vi "Load Plugin.vi"(6 "timeout (ms)":i32=5000, 8 "error in":errorcluster, 9 "Plugin Path":string, 10 "Plugin Name":string, 11 "gRPC ID in":T1) -> (0 "error out":errorcluster, 3 "gRPC ID out":T1)   [LabVIEW 2021, in "CIFPluginLoaderClientWrapper.lvlib"]
uses:
  CIFPluginLoaderClientWrapper.lvlib
  <vilib>/gRPC/LabVIEW gRPC Library/Shared/grpcId.ctl
  CIF_PluginLoader_client/RPC Messages/cif_pluginloader_LoadPluginRequest.ctl
  CIF_PluginLoader_client/CIF_PluginLoader_client.lvlib
  <vilib>/gRPC/LabVIEW gRPC Library/grpc-lvsupport-release.lvlib
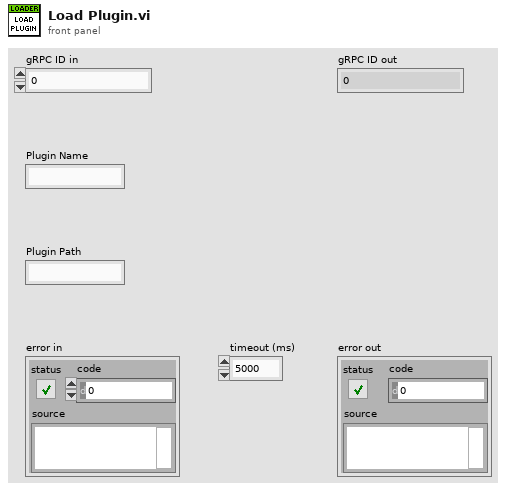
[diagram p1: front panel]
types:
  T1 = typedef "grpc-lvsupport-release.lvlib/grpcId.ctl" = u64
  T2 = typedef "CIF_PluginLoader_client.lvlib/cif_pluginloader_LoadPluginRequest.ctl" = cluster{"plugin_name":string, "path":string}
  T3 = typedef "CIF_PluginLoader_client.lvlib/cif_pluginloader_LoadPluginResponse.ctl" = cluster{"status":T4}
  T4 = typedef "CIF_PluginLoader_client.lvlib/cif_common_Status.ctl" = cluster{"code":i32, "message":string}
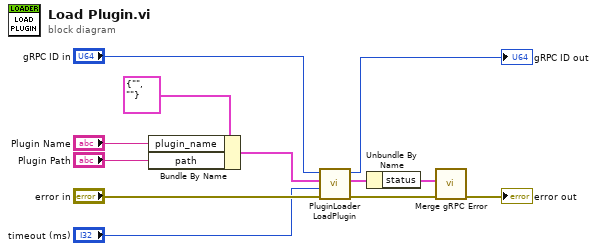
[diagram p0: block diagram]
diagram:
  n1 = Bundle By Name(cluster=T2 {"plugin_name"="", "path"=""} ("Request Data"), "plugin_name"="Plugin Name", "path"="Plugin Path") -> (w3:T2)
  n2 = call "PluginLoader LoadPlugin.vi"("error in"="error in", "timeout (ms)"="timeout (ms)", "Request Data"=w3, "gRPC ID"="gRPC ID in") -> ("error out"=w8:errorcluster, "Response Data"=w6:T3, "gRPC ID out"=→"gRPC ID out":T1)  [unwired: 5 in]
  n3 = Unbundle By Name(w6) -> ("status"=w1:T4)
  n4 = call "Merge gRPC Error.vi"("error in (no error)"=w8, "gRPC Error"=w1) -> ("error out"=→"error out":errorcluster)  [unwired: 9 in]
